vi "Helper SubVI - Adjust Phase.vi"(11 "Phase":dbl[](array[numeric])) -> (3 "Adjusted phase":dbl[](array[numeric]))   [LabVIEW 2023]
doc: "Adjusts the phase of the selected mode."
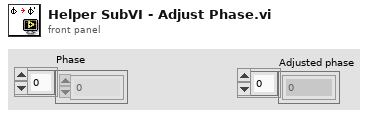
[diagram p1: front panel]
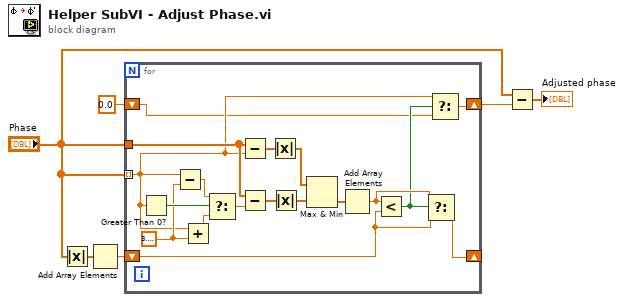
[diagram p0: block diagram]
diagram:
  n1 = Absolute Value(x="Phase") -> (abs(x)=w6:dbl[])
  n2 = Add Array Elements(numeric array=w6) -> (sum=w5:dbl)
  n3 = for {
    tunnel: "Phase" -> [w10] mode=indexing
    tunnel: "Phase" -> [w19]
    shift-right: [w12] -> _
    shift-left: w5 -> [w13]
    shift-right: [w8] -> w3
    shift-left: 0.0 ("Numeric") -> [w9]
    w22 = 3.141592653589793 ("Pi")
    n4 = Greater Than 0?(x=w10) -> (x > 0?=w24:bool)
    n5 = Subtract(x=w10, y=w22) -> (x-y=w23:dbl)
    n6 = Add(x=w10, y=w22) -> (x+y=w21:dbl)
    n7 = Select(t=w23, s=w24, f=w21) -> (s? t:f=w20:dbl)
    n8 = Subtract(x=w19, y=w10) -> (x-y=w7:dbl[])
    n9 = Subtract(x=w19, y=w20) -> (x-y=w18:dbl[])
    n10 = Absolute Value(x=w7) -> (abs(x)=w17:dbl[])
    n11 = Absolute Value(x=w18) -> (abs(x)=w16:dbl[])
    n12 = Max & Min(x=w17, y=w16) -> (min(x,y)=w15:dbl[])  [unwired: 1 out]
    n13 = Add Array Elements(numeric array=w15) -> (sum=w14:dbl)
    n14 = Less?(x=w14, y=w13) -> (x < y?=w11:bool)
    n15 = Select(t=w14, s=w11, f=w13) -> (s? t:f=w12:dbl)
    n16 = Select(t=w10, s=w11, f=w9) -> (s? t:f=w8:dbl)
  }
  n17 = Subtract(x="Phase", y=w3) -> (x-y=→"Adjusted phase":dbl[])
